vi "Read State Class.vi"(8 "error in (no error)":errorcluster, 11 "DAQ Controller in":refnum<class "DAQ Controller.lvclass">) -> (0 "error out":errorcluster, 2 "Process State Data":refnum<data-value>, 3 "DAQ Controller out":refnum<class "DAQ Controller.lvclass">)   [LabVIEW 2022 SP3, in "DAQ Controller.lvclass"]
uses:
  DAQ Controller.lvclass
  XY Stage/Process Actor/Process Framework/Process State Data/Process State Data.lvclass
  DAQ Controller.lvclass/DAQ Controller.ctl
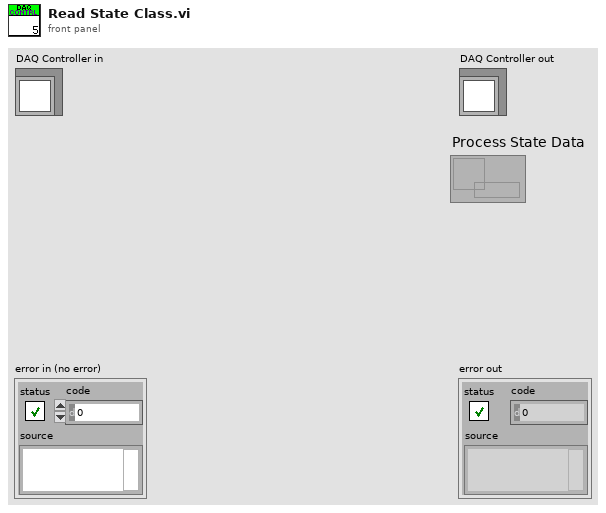
[diagram p1: front panel]
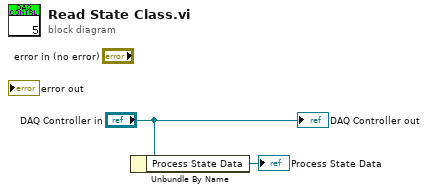
[diagram p0: block diagram]
diagram:
  n1 = Unbundle By Name("DAQ Controller in") -> ("Process State Data"=→"Process State Data":refnum<data-value>)
  "DAQ Controller out" <- "DAQ Controller in"
